vi "FlatToRichni_measurementlink_pinmap_v1_QueryPinsRequest.vi"(5 "OutputClusterType":T1, 11 "InputCluster":T2) -> (3 "OutputCluster":T1)   [LabVIEW 2020, in "Measurement Plugin Pin Map Client.lvlib"]
uses:
  Measurement Plugin Pin Map Client.lvlib
  ni_measurementlink_pinmap_v1_QueryPinsRequest_Flat.ctl
  ni_measurementlink_pinmap_v1_QueryPinsRequest.ctl
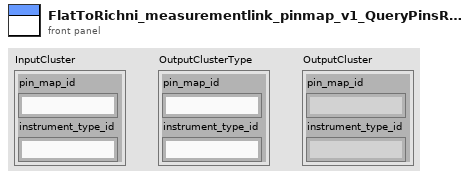
[diagram p1: front panel]
types:
  T1 = typedef "Measurement Plugin Pin Map Client.lvlib/ni_measurementlink_pinmap_v1_QueryPinsRequest.ctl" = cluster{"pin_map_id":string, "instrument_type_id":string}
  T2 = typedef "Measurement Plugin Pin Map Client.lvlib/ni_measurementlink_pinmap_v1_QueryPinsRequest_Flat.ctl" = cluster{"pin_map_id":string, "instrument_type_id":string}
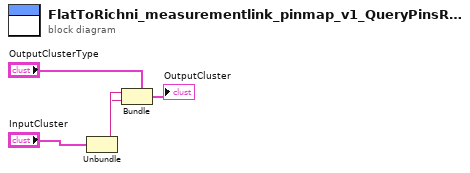
[diagram p0: block diagram]
diagram:
  n1 = Unbundle "Unbundle"("InputCluster") -> ("pin_map_id"=w2:string, "instrument_type_id"=w1:string)
  n2 = Bundle "Bundle"(cluster="OutputClusterType", "pin_map_id"=w2, "instrument_type_id"=w1) -> (→"OutputCluster":T1)
